vi "Aliasing 3.vi"() -> ()   [LabVIEW 2017]
panel:
  in  "stop":bool
  out "Waveform Graph":waveform(dbl)[](graph)=[{"t0"=timestamp(0 s since 1904-01-01), "dt"=0.025000000000000005, "Y"=array[400 elements]}, {"t0"=timestamp(0 s since 1904-01-01), "dt"=1.0, "Y"=[0.7071067811865476, -0.4539904997395467, -0.9876883405951378, -0.15643446504023192, 0.8910065241883673, 0.7071067811865483, -0.45399049973954414, -0.9876883405951382, -0.15643446504023392, 0.8910065241883665]}, {"t0"=timestamp(0 s since 1904-01-01), "dt"=0.025000000000000005, "Y"=array[400 elements]}, {"t0"=timestamp(0 s since 1904-01-01), "dt"=0.025000000000000005, "Y"=array[400 elements]}]
  in  "Tab Control":enum32{"Hovedside", "Innstillinger"}(tab)
  in  "Visible":bool[](array[boolean])=[TRUE, FALSE, FALSE]
  in  "Frekvenser":dbl[](array[numeric])=[0.19999999999999996, 1.2, -0.2] step=0.1
  in  "Fase [Grader]":dbl=45.0
  in  "Perioder":i32=2
  in  "fm color":u32(colorbox)=16711680
  in  "f0 color":u32(colorbox)=16448250
  in  "fk color":u32(colorbox)=16777224
  # "Sampling og Aliasing"
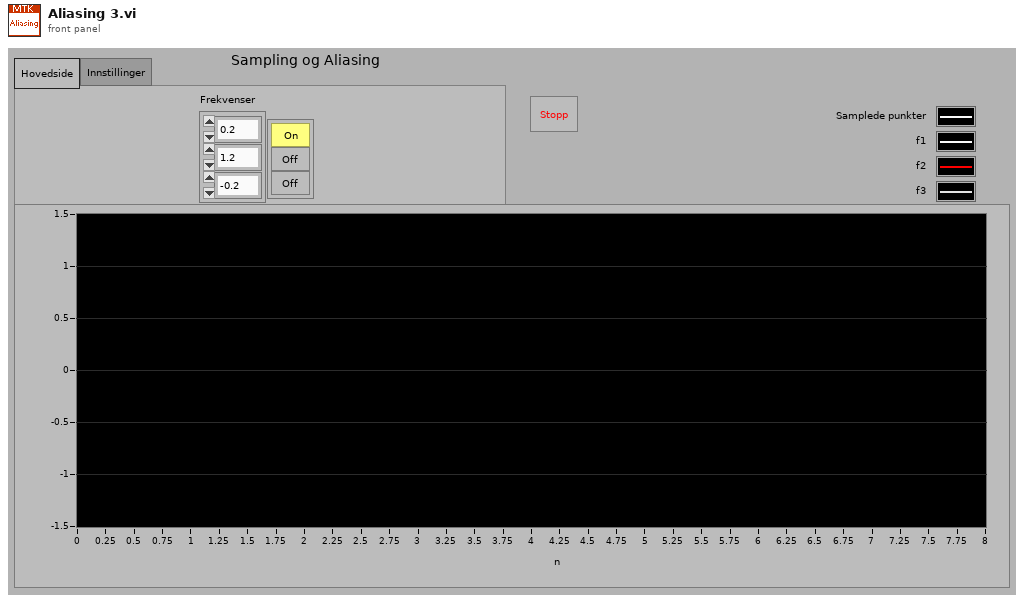
[diagram p1: front panel]
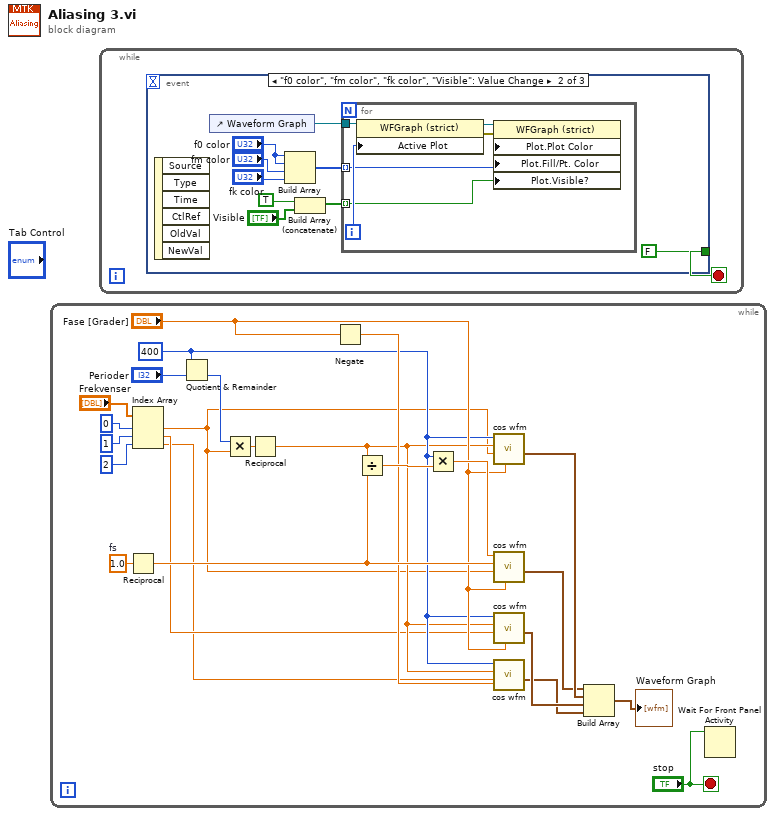
[diagram p0: block diagram]
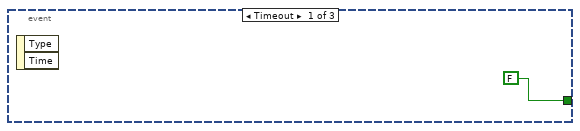
[diagram p2: hidden frame]
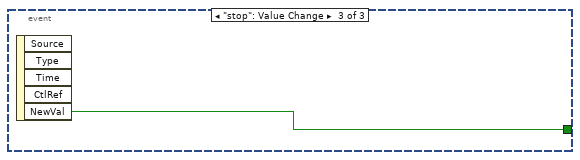
[diagram p3: hidden frame]
diagram:
  n1 = while {
    stop <- "stop" stop-if-true
    w12 = 1.0  # fs
    w16 = 400 ("samples")
    n2 = Reciprocal(x=w12) -> (1/x=w22:dbl)
    n3 = Index Array(array="Frekvenser", index #1=0, index #2=1, index #3=2) -> (element #1=w3:dbl, element #2=w2:dbl, element #3=w1:dbl)
    n4 = Quotient & Remainder(x=w16, y="Perioder") -> (floor(x/y)=w14:i32)  [unwired: 1 out]
    n5 = Multiply(x=w14, y=w3) -> (x*y=w17:dbl)
    n6 = Reciprocal(x=w17) -> (1/x=w13:dbl)
    n7 = Negate(x="Fase [Grader]") -> (-x=w18:dbl)
    n8 = Divide(x=w13, y=w22) -> (x/y=w21:dbl)
    n9 = Multiply(x=w16, y=w21) -> (x*y=w20:dbl)
    n10 = call "cos wfm.vi"("phi"="Fase [Grader]", "f"=w3, "dt"=w13, "N"=w16) -> ("cos wt"=w24:waveform(dbl))  [unwired: 7 out]
    n11 = call "cos wfm.vi"("phi"="Fase [Grader]", "f"=w3, "dt"=w22, "N"=w20) -> ("cos wt"=w8:waveform(dbl))  [unwired: 7 out]
    n12 = call "cos wfm.vi"("phi"="Fase [Grader]", "f"=w2, "dt"=w13, "N"=w16) -> ("cos wt"=w11:waveform(dbl))  [unwired: 7 out]
    n13 = call "cos wfm.vi"("phi"=w18, "f"=w1, "dt"=w13, "N"=w16) -> ("cos wt"=w10:waveform(dbl))  [unwired: 7 out]
    n14 = Build Array(w8, w24, w11, w10) -> (→"Waveform Graph":waveform(dbl)[])
    n15 = Wait For Front Panel Activity(3:"stop") -> ()  [unwired: 3 out]
  }
  n16 = while {
    stop <- w25 stop-if-true
    n17 = event shown="[1] \"f0 color\", \"fm color\", \"fk color\", \"Visible\": Value Change" {
      selector: _ -> [_ _ _]
      dyn-events: _ -> [_ _ _]
      timeout: _ -> [_ _ _]
      tunnel: [FALSE ("NewVal") FALSE ("NewVal") w42] -> w25
      event Timeout {
        n18 = event-data() -> ()  [unwired: 3 out]
      }
      event "f0 color", "fm color", "fk color", "Visible": Value Change {
        n19 = event-data() -> ()  [unwired: 7 out]
        n20 = control-ref of="Waveform Graph"() -> (w31:refnum<vi>)
        n21 = Build Array("f0 color", "f0 color", "fm color", "fk color") -> (w32:u32[])
        n22 = Build Array (concatenate)(TRUE ("f3 2"), "Visible") -> (w28:bool[])
        n23 = for {
          tunnel: w32 -> [w37] mode=indexing
          tunnel: w31 -> [w41]
          tunnel: w28 -> [w36] mode=indexing
          i -> [w38]
          n24 = property class="WFGraph (strict)"(reference=w41, "Active Plot"=w38) -> (reference out=w40:refnum<vi>, error out=w39:errorcluster)  [unwired: 1 in]
          n25 = property class="WFGraph (strict)"(reference=w40, error in=w39, "Plot.Plot Color"=w37, "Plot.Fill/Pt. Color"=w37, "Plot.Visible?"=w36) -> ()  [unwired: 2 out]
        }
      }
      event "stop": Value Change {
        n26 = event-data() -> ("NewVal"=w42:bool)  [unwired: 5 out]
      }
    }
  }
